vi "labview播放mp4檔案__8_24.vi"() -> ()   [LabVIEW 2019]
panel:
  in  "stop":bool
  in  "Path":path
  in  "WindowsMediaPlayer":refnum<k7>(container)
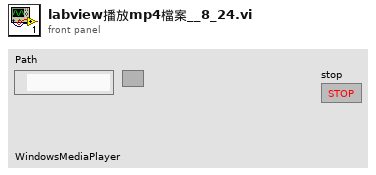
[diagram p1: front panel]
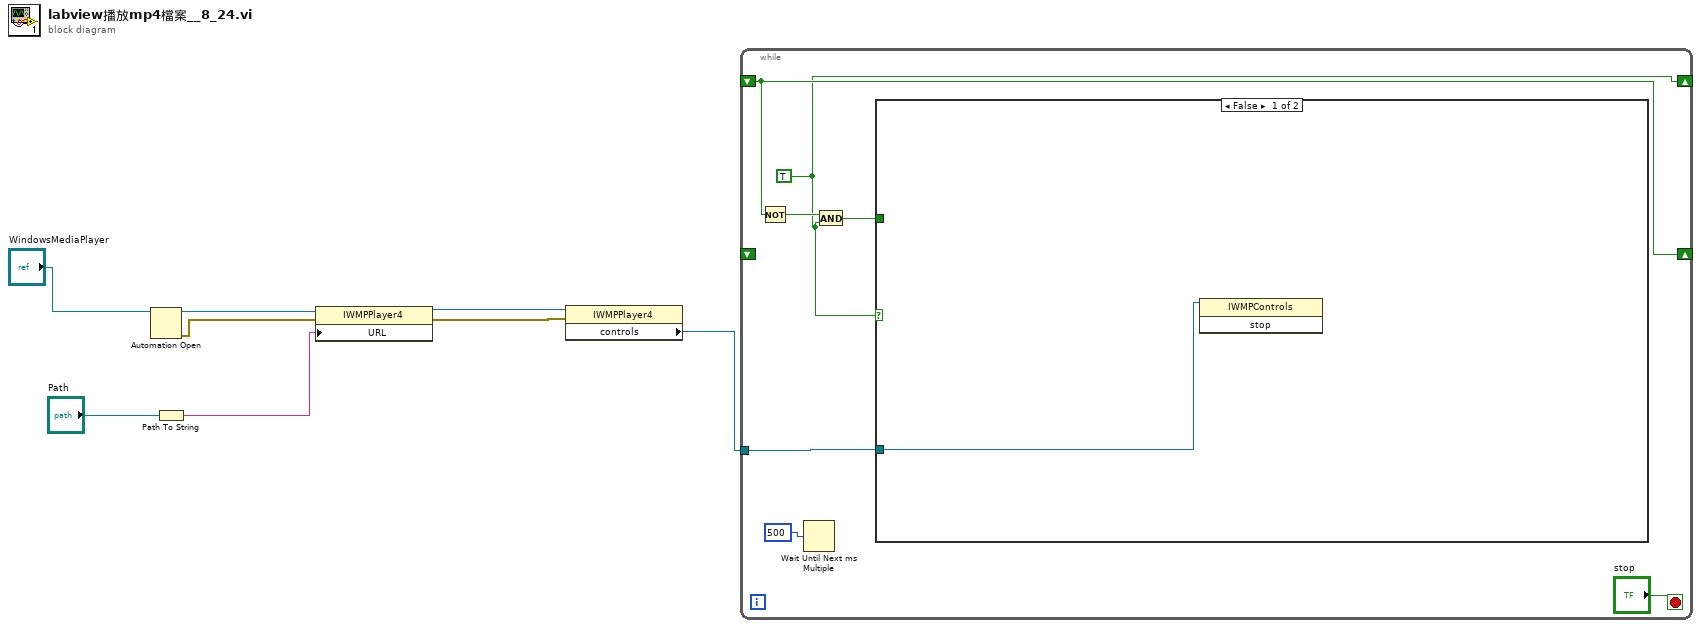
[diagram p0: block diagram]
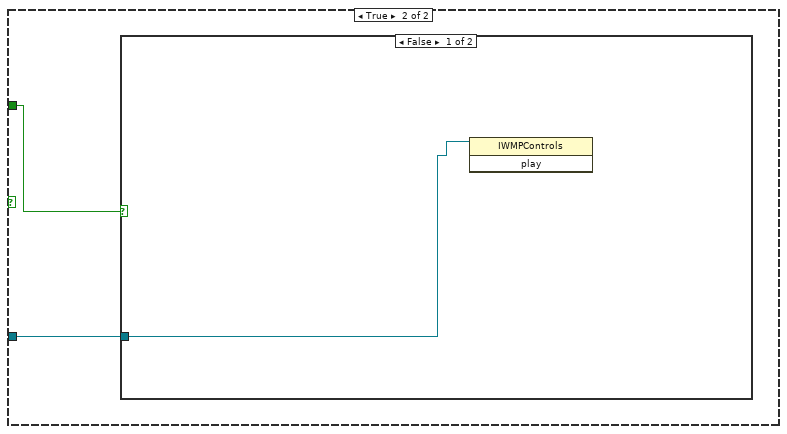
[diagram p2: hidden frame]
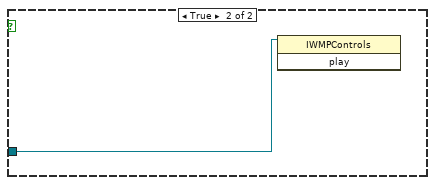
[diagram p3: hidden frame]
diagram:
  n1 = Automation Open(Automation Refnum="WindowsMediaPlayer") -> (Automation Refnum=w3:refnum<k7>, error out=w5:errorcluster)  [unwired: 3 in]
  n2 = Path To String(path="Path") -> (string=w7:string)
  n3 = property class="IWMPPlayer4"(reference=w3, error in=w5, "URL"=w7) -> (reference out=w4:refnum<k7>, error out=w6:errorcluster)
  n4 = property class="IWMPPlayer4"(reference=w4, error in=w6) -> ("controls"=w1:refnum<k7>)  [unwired: 2 out]
  n5 = while {
    tunnel: w1 -> [w14]
    shift-right: [w10] -> _
    shift-left: _ -> [_]
    shift-right: [w9] -> _
    shift-left: _ -> [w10]
    stop <- "stop" stop-if-true
    w9 = TRUE
    n6 = Not(x=w10) -> (.not. x?=w13:bool)
    n7 = Wait Until Next ms Multiple(millisecond multiple=u32 500 ("millisecond timer value")) -> ()  [unwired: 1 out]
    n8 = And(x=w13, y=w9) -> (x .and. y?=w12:bool)
    n9 = case shown="False" w9 {
      tunnel: w14 -> [w16 w18]
      tunnel: w12 -> [_ w17]
      frame False {
        n10 = invoke class="IWMPControls" method="stop"(reference=w16) -> ()  [unwired: 2 in, 3 out]
      }
      frame True {
        n11 = case shown="False" w17 {
          tunnel: w18 -> [w19 w20]
          frame False {
            n12 = invoke class="IWMPControls" method="play"(reference=w19) -> ()  [unwired: 2 in, 3 out]
          }
          frame True {
            n13 = invoke class="IWMPControls" method="play"(reference=w20) -> ()  [unwired: 2 in, 3 out]
          }
        }
      }
    }
  }
